vi "Scripting_LVClassScriptingProps.vi"() -> ()   [LabVIEW 2016]
panel:
  in  "LVClassLibrary Refnum":refnum<vi>
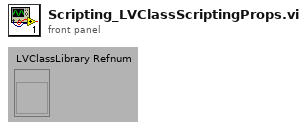
[diagram p1: front panel]
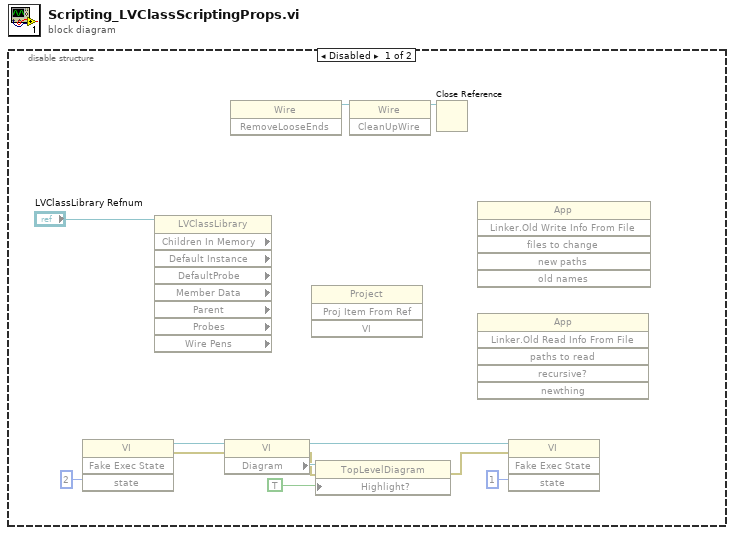
[diagram p0: block diagram]
diagram:
  n1 = disable-structure shown="Disabled" {
    frame Disabled {
      n2 = invoke class="VI" method="Fake Exec State"("state"=2 ("State")) -> (reference out=w10:refnum<vi>, error out=w9:errorcluster)  [unwired: 3 in, 2 out]
      n3 = property class="LVClassLibrary" props=["Children In Memory", "Default Instance", "DefaultProbe", "Member Data", "Parent", "Probes", "Wire Pens"](reference="LVClassLibrary Refnum") -> ()  [unwired: 1 in, 9 out]
      n4 = property class="VI"(reference=w10, error in=w9) -> (reference out=w7:refnum<vi>, error out=w8:errorcluster, "Diagram"=w11:refnum<vi>)
      n5 = invoke class="Wire" method="RemoveLooseEnds"() -> (reference out=w2:refnum<vi>)  [unwired: 3 in, 2 out]
      n6 = invoke class="Project" method="Proj Item From Ref"() -> ()  [unwired: 4 in, 4 out]
      n7 = property class="TopLevelDiagram"(reference=w11, error in=w8, "Highlight?"=TRUE) -> (error out=w6:errorcluster)  [unwired: 1 out]
      n8 = invoke class="Wire" method="CleanUpWire"(reference=w2) -> (reference out=w1:refnum<vi>)  [unwired: 2 in, 2 out]
      n9 = Close Reference(reference=w1) -> ()  [unwired: 1 in, 1 out]
      n10 = invoke class="App" method="Linker.Old Write Info From File"() -> ()  [unwired: 6 in, 6 out]
      n11 = invoke class="App" method="Linker.Old Read Info From File"() -> ()  [unwired: 6 in, 6 out]
      n12 = invoke class="VI" method="Fake Exec State"(reference=w7, error in=w6, "state"=1 ("State")) -> ()  [unwired: 1 in, 4 out]
    }
    frame Enabled {
    }
  }
